vi "struct_ads_vol_w_pTpsatRho.vi"(5 "Saturated liquid density of adsorpt in kg/m3 (Input)":dbl, 7 "Saturation pressure in Pa (Input)":dbl, 8 "Error (Input)":errorcluster, 9 "Temperature in K (Input)":dbl, 10 "Pressure in Pa (Input)":dbl, 11 "Reference working pair (Input)":i64) -> (0 "Error (Output)":errorcluster caption="Error(Output)", 3 "Loading in kg/kg (Output)":dbl)   [LabVIEW 2017]
doc: "ads_vol_w_pTpsatRho:\n * --------------------\n *\n * Calculates equilibrium loading w in kg/kg depending on equilibrium pressure\n * p in Pa, equilibrium temperature T in K, saturation pressure p_Sat in Pa and\n * saturated liquid density of adsorpt rho in kg/m³.\n *\n * Parameters:\n * -----------\n * double p_Pa:\n * Equilibrium pressure in Pa.\n * double T_K:\n * Equilibrium temperature in K.\n * double p_sat_Pa:\n * Saturation pressure in Pa.\n * double rho_l_kgm3:\n * Saturated liquid density of adsorpt in kg/m³.\n * struct *WorkingPair:\n * Pointer of WorkingPair-struct.\n *\n * Returns:\n * --------\n * double:\n * Equilibrium loading in kg/kg.\n *\n * History:\n * --------\n * 07/13/2021, by Jannik Driesel (supervised by Mirko Engelpracht):\n * First implementation."
uses:
  data/win32bit/libsorpPropLib.dll
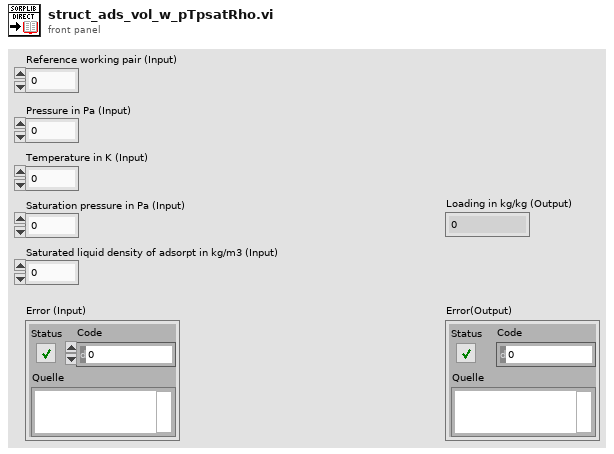
[diagram p1: front panel]
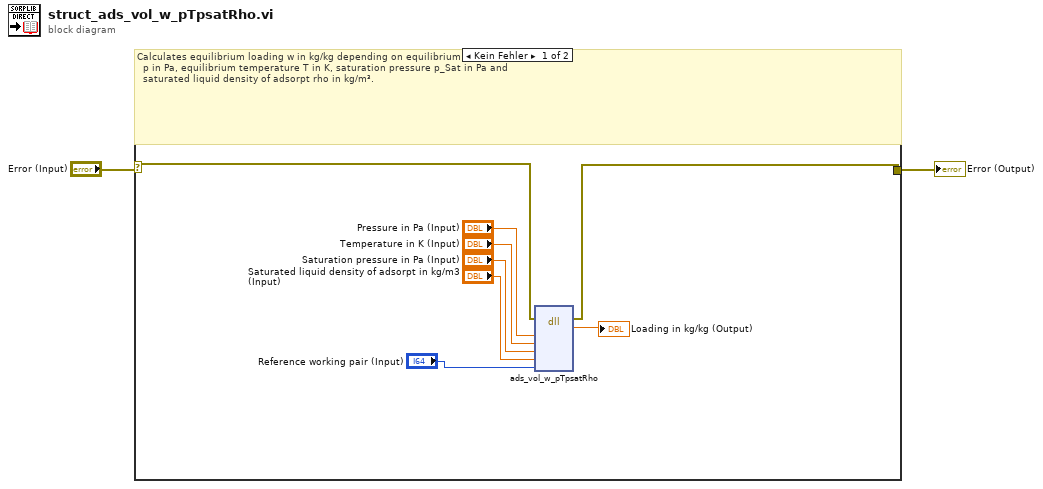
[diagram p0: block diagram]
diagram:
  n1 = case shown="Kein Fehler" "Error (Input)" {
    selector: "Error (Input)" -> [w9 w11]
    tunnel: [w8 w11] -> w1
    frame No Error {
      # "Calculates equilibrium loading w in kg/kg depending on equilibrium pressure\n  p in Pa, equilibrium temperature T in K, saturation pressure p_Sat in Pa and\n  saturated liquid density of adsorpt rho in kg/m³."
      n2 = dll-call lib="D:/Driesel/SorpLibLocal/LabVIEW_wrapper/data/win32bit/libsorpPropLib.dll" fn="ads_vol_w_pTpsatRho"(error in=w9, "p_Pa"="Pressure in Pa (Input)", "T_K"="Temperature in K (Input)", "p_sat_Pa"="Saturation pressure in Pa (Input)", "rho_l_kgm3"="Saturated liquid density of adsorpt in kg/m3 (Input)", "workingPair"="Reference working pair (Input)") -> (error out=w8:errorcluster, "w_kgkg"=→"Loading in kg/kg (Output)":dbl)  [unwired: 7 in, 1 out]
    }
    frame Error {
      # "Error - No calculations"
    }
  }
  "Error (Output)" <- w1
